vi "Cage-connect.vi"(8 "error in (no error)":errorcluster, 9 "Cluster in":T1={"Position"=0.0, "Is.Enabled?"=FALSE, "Is.Connected?"=FALSE, "Device SN"="45876539", "AccelerationMaximum"=0.0, "VelocityMaximum"=0.0, "Acceleration"=0.0, "Velocity"=0.0, "waitTimeout (ms)"=0, "Model"=enum."None", "Is.Homed?"=FALSE}, 11 "reference in":refnum<k24>) -> (0 "error out":errorcluster, 1 "Cluster out":T1={"Position"=0.0, "Is.Enabled?"=FALSE, "Is.Connected?"=FALSE, "Device SN"="45876539", "AccelerationMaximum"=0.0, "VelocityMaximum"=0.0, "Acceleration"=0.0, "Velocity"=0.0, "waitTimeout (ms)"=0, "Model"=enum."None", "Is.Homed?"=FALSE}, 2 "IsConnected":bool, 3 "reference out":refnum<k24>)   [LabVIEW 2018]
uses:
  C:/Project/SerialSectionOCT/SerialSectOCT/Labview Software/Thorlabs.MotionControl.Controls.dll
  Thorlabs.MotionControl.Controls.dll
  Thorlabs Translation Stages/Controls/Translation Stage Cluster.ctl
  General/Controls/Translation Stage Types.ctl
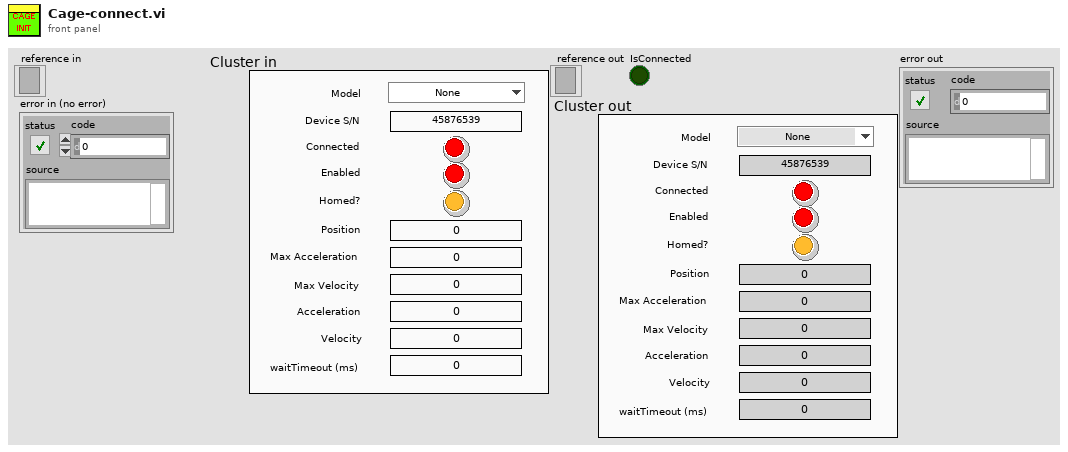
[diagram p1: front panel]
types:
  T1 = typedef "Translation Stage Cluster.ctl" = cluster{"Position":dbl, "Is.Enabled?":bool, "Is.Connected?":bool, "Device SN":string, "AccelerationMaximum":dbl, "VelocityMaximum":dbl, "Acceleration":dbl, "Velocity":dbl, "waitTimeout (ms)":i32, "Model":T2, "Is.Homed?":bool}
  T2 = typedef "Translation Stage Types.ctl" = enum16{"None", "Thorlabs LTS", "Thorlabs MLJ"}
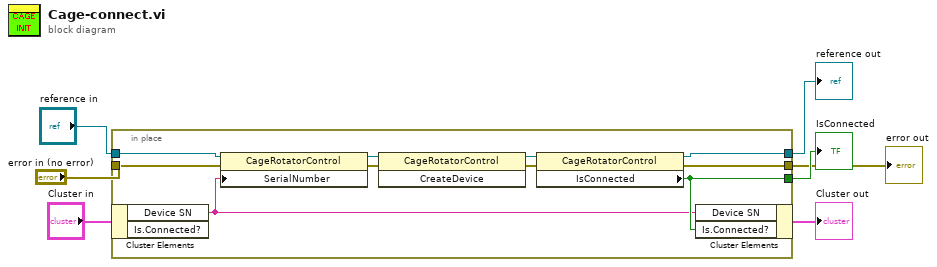
[diagram p0: block diagram]
diagram:
  n1 = in-place {
    in-place-border: "reference in" -> [w15]
    in-place-border: [w12] -> w3
    in-place-border: "error in (no error)" -> [w11]
    in-place-border: [w10] -> w1
    in-place-border: [w9] -> w2
    n2 = in-place-cluster #1("Cluster in") -> ("Device SN"=w8:string)  [unwired: 1 out]
    n3 = property class="CageRotatorControl"(reference=w15, error in=w11, "SerialNumber"=w8) -> (reference out=w17:refnum<k24>, error out=w16:errorcluster)
    n4 = invoke class="CageRotatorControl" method="CreateDevice"(reference=w17, error in=w16) -> (reference out=w14:refnum<k24>, error out=w13:errorcluster)  [unwired: 1 in, 1 out]
    n5 = property class="CageRotatorControl"(reference=w14, error in=w13) -> (reference out=w12:refnum<k24>, error out=w10:errorcluster, "IsConnected"=w9:bool)
    n6 = in-place-cluster #1("Device SN"=w8, "Is.Connected?"=w9) -> (→"Cluster out":T1)
  }
  "reference out" <- w3
  "IsConnected" <- w2
  "error out" <- w1
